vi "Variable Graphing.vi"(0 "Tree Refnum":refnum<vi>) -> ()   [LabVIEW 2017]
uses:
  <vilib>/Utility/miscctls.llb/LVRangeTypeDef.ctl
  <vilib>/Platform/TimedLoop/XDataNode/timing_clust.ctl
  <vilib>/Platform/TimedLoop/XDataNode/nitl_modes.ctl
  <vilib>/Platform/TimedLoop/XDataNode/wakeup.ctl
  <vilib>/Rock Robotics/Network Tables/NT Read Number.vi
  <vilib>/Rock Robotics/Network Tables/NT Write Number.vi
  <vilib>/Rock Robotics/Network Tables/NT Write Boolean.vi
  <vilib>/platform/TimedLoop/XDataNode/XDataNode.xnode
  <vilib>/Platform/TimedLoop/XDataNode/XDNodeRunTimeDep.lvlib
panel:
  in  "Camera Tab":enum32{"Graphs Setup", "PID Test", "Variables"}(tab)
  in  "Graph 2 Variable Selection":T1
  in  "Graph 1 Variable Selection":T2
  in  "Graph Include Filter":string[](array[string])
  in  "Graph Exclude Filter":string[](array[string])
  in  "Chart Update Rate Samples":i32=10
  in  "Waveform Depth Samples":i32=6000
  out "Chart":waveform(dbl)[](graph)
  out "Chart 2":waveform(dbl)[](graph)
  out "Samples":i32
  in  "Reset":bool
  in  "Pause":bool
  in  "Talon Performance Values":u16(ring) items=["/Talons/1/Bus Voltage", "/Talons/1/Closed Loop Error", "/Talons/1/Error Derivative", "/Talons/1/Integral Acummulator", "/Talons/1/Output Current", "/Talons/1/Output Voltage", "/Talons/1/Percent Output", "/Talons/1/Position", "/Talons/1/Velocity", "/Talons/1/pid:0/D", "/Talons/1/pid:0/FF", "/Talons/1/pid:0/I", "/Talons/1/pid:0/IZone", "/Talons/1/pid:0/P", "/Talons/1/pid:1/D", "/Talons/1/pid:1/FF", "/Talons/1/pid:1/I", "/Talons/1/pid:1/IZone", "/Talons/1/pid:1/P", "/Talons/2/Bus Voltage", "/Talons/2/Closed Loop Error", "/Talons/2/Error Derivative", "/Talons/2/Integral Acummulator", "/Talons/2/Output Current", "/Talons/2/Output Voltage", "/Talons/2/Percent Output", "/Talons/2/Position", "/Talons/2/Velocity", "/Talons/2/pid:0/D", "/Talons/2/pid:0/FF", "/Talons/2/pid:0/I", "/Talons/2/pid:0/IZone", "/Talons/2/pid:0/P", "/Talons/2/pid:1/D", "/Talons/2/pid:1/FF", "/Talons/2/pid:1/I", "/Talons/2/pid:1/IZone", "/Talons/2/pid:1/P", "/Talons/3/Bus Voltage", "/Talons/3/Closed Loop Error", "/Talons/3/Error Derivative", "/Talons/3/Integral Acummulator", "/Talons/3/Output Current", "/Talons/3/Output Voltage", "/Talons/3/Percent Output", "/Talons/3/Position", "/Talons/3/Velocity", "/Talons/3/pid:0/D", "/Talons/3/pid:0/FF", "/Talons/3/pid:0/I", "/Talons/3/pid:0/IZone", "/Talons/3/pid:0/P", "/Talons/3/pid:1/D", "/Talons/3/pid:1/FF", "/Talons/3/pid:1/I", "/Talons/3/pid:1/IZone", "/Talons/3/pid:1/P", "/Talons/4/Bus Voltage", "/Talons/4/Closed Loop Error", "/Talons/4/Error Derivative", "/Talons/4/Integral Acummulator", "/Talons/4/Output Current", "/Talons/4/Output Voltage", "/Talons/4/Percent Output", "/Talons/4/Position", "/Talons/4/Velocity", "/Talons/4/pid:0/D", "/Talons/4/pid:0/FF", "/Talons/4/pid:0/I", "/Talons/4/pid:0/IZone", "/Talons/4/pid:0/P", "/Talons/4/pid:1/D", "/Talons/4/pid:1/FF", "/Talons/4/pid:1/I", "/Talons/4/pid:1/IZone", "/Talons/4/pid:1/P"]
  in  "Talon Array":T3(array[cluster])
  in  "Run Selected":bool
  in  "Set Point":dbl
  in  "Read All":bool
  in  "Update\nSelected":bool
  in  "Talon ID Selector":u16(ring) items=["1", "2", "3", "4"]
  out "Chart 3":waveform(dbl)[](graph)
  in  "Pause PID":bool
  in  "Reset PID":bool
  out "Samples 2":i32
  in  "Waveform Depth Samples 2":i32=6000
  in  "Chart Update Rate Samples 2":i32=10
  out "Tree":string(tree)
  # "Graph 1"
  # "Graph 2"
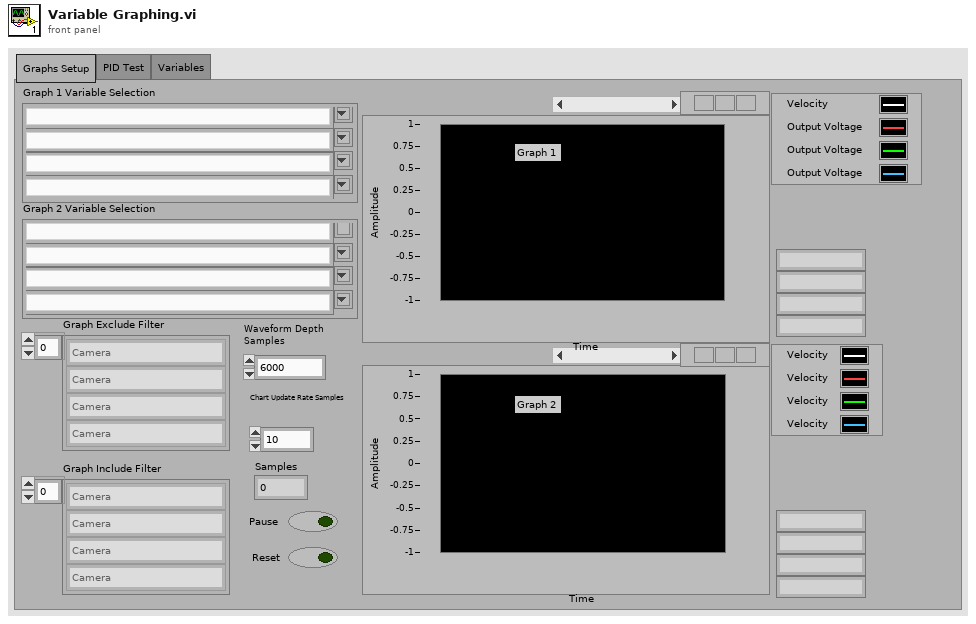
[diagram p1: front panel]
types:
  T1 = cluster{"Combo Box 5":string, "Combo Box 6":string, "Combo Box 7":string, "Combo Box 8":string}
  T2 = cluster{"Combo Box":string, "Combo Box 2":string, "Combo Box 3":string, "Combo Box 4":string}
  T3 = cluster{"P":dbl, "I":dbl, "D":dbl, "FF":dbl, "IZone":dbl, "RR":dbl, "Mode":dbl}[][]
  T4 = cluster{"P":dbl, "I":dbl, "D":dbl, "FF":dbl, "IZone":dbl, "RR":dbl, "Mode":dbl}
  T5 = typedef "LVRangeTypeDef.ctl" = cluster{"Minimum":dbl, "Maximum":dbl, "Increment":dbl, "Minor Increment":dbl, "Start":dbl}
  T6 = typedef "XDNodeRunTimeDep.lvlib/timing_clust.ctl" = cluster{"Expected End [f-1]":u64, "Actual End [f-1]":u64, "Finished Late? [f-1]":bool, "Expected End [i-1]":u64, "Actual End [i-1]":u64, "Finished Late? [i-1]":bool, "Expected Start [i]":u64, "Actual Start [i]":u64, "Expected Start [f]":u64, "Actual Start [f]":u64, "Source Name":string, "Structure Name":string, "Period":i64, "Deadline":i64, "Offset":i64, "Start":i64, "Priority":i32, "Timeout":i32, "Mode":T7, "Wakeup Reason":T8, "Error":errorcluster, "Source Type":string, "Secondary Source Type":string, "Global End Time":u64, "Global Start Time":u64, "Frame Duration":u64, "Iteration Duration":u64, "Assigned CPU":i32, "I/O Scan Engine Mode":u32}
  T7 = typedef "XDNodeRunTimeDep.lvlib/nitl_modes.ctl" = enum32{"No Change", "Process missed periods, maintain original phase", "Discard missed periods, maintain original phase", "Process missed periods, ignore original phase", "Discard missed periods, ignore original phase"}
  T8 = typedef "XDNodeRunTimeDep.lvlib/wakeup.ctl" = enum32{"Normal", "Aborted", "Asynchronous wakeup", "Timing source error", "Timed loop error", "Timeout"}
  T9 = cluster{"P":dbl, "I":dbl, "D":dbl, "FF":dbl, "IZone":dbl, "RR":dbl, "Mode":dbl}[]
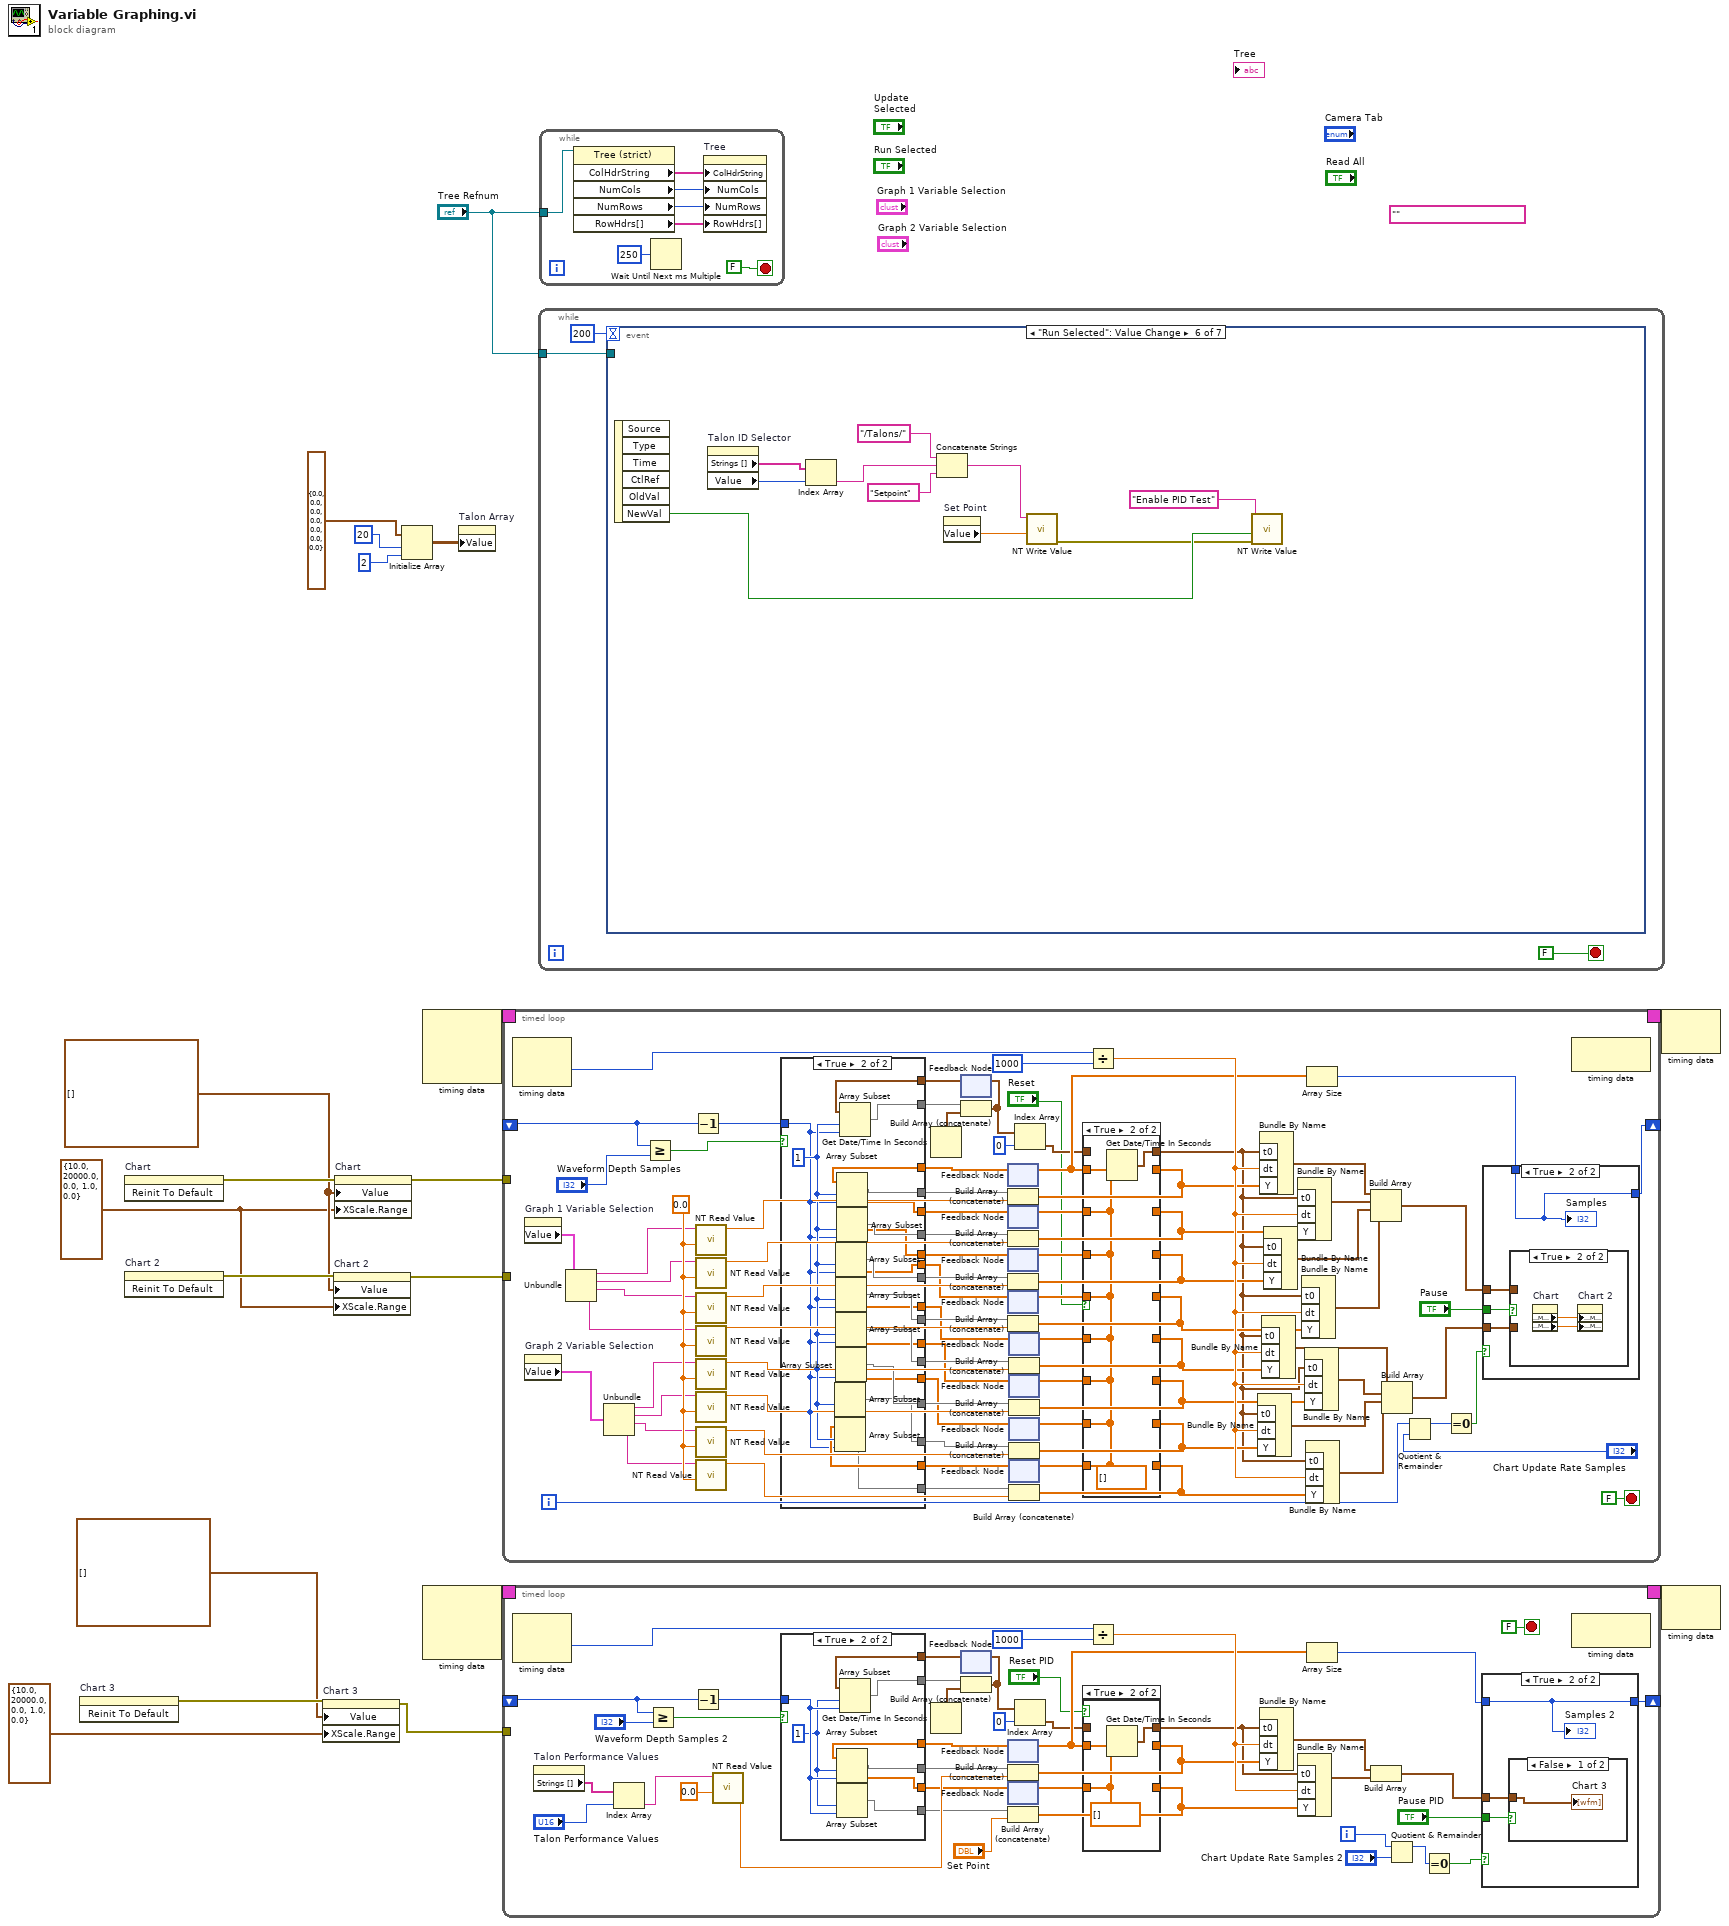
[diagram p0: block diagram]
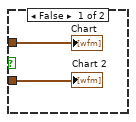
[diagram p8: hidden frame]
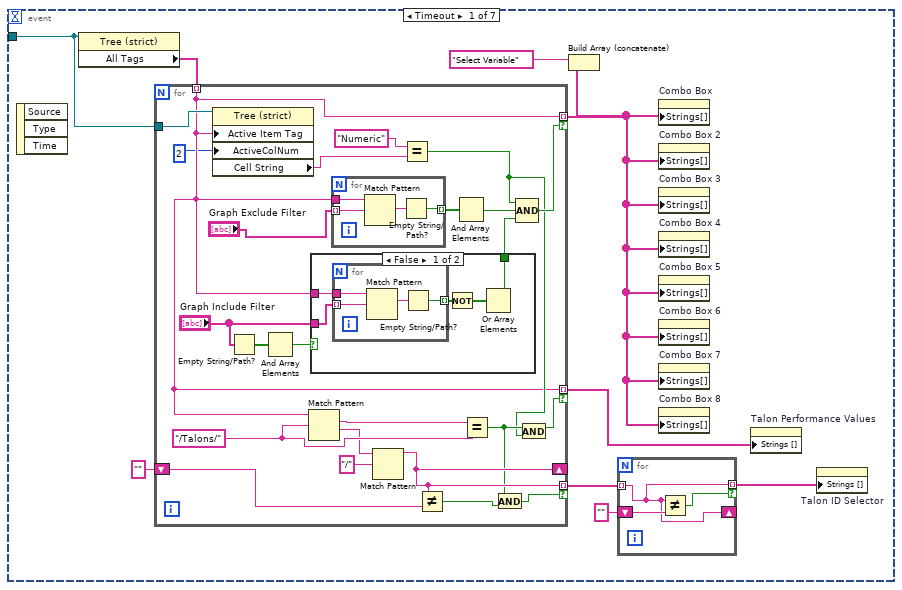
[diagram p10: hidden frame]
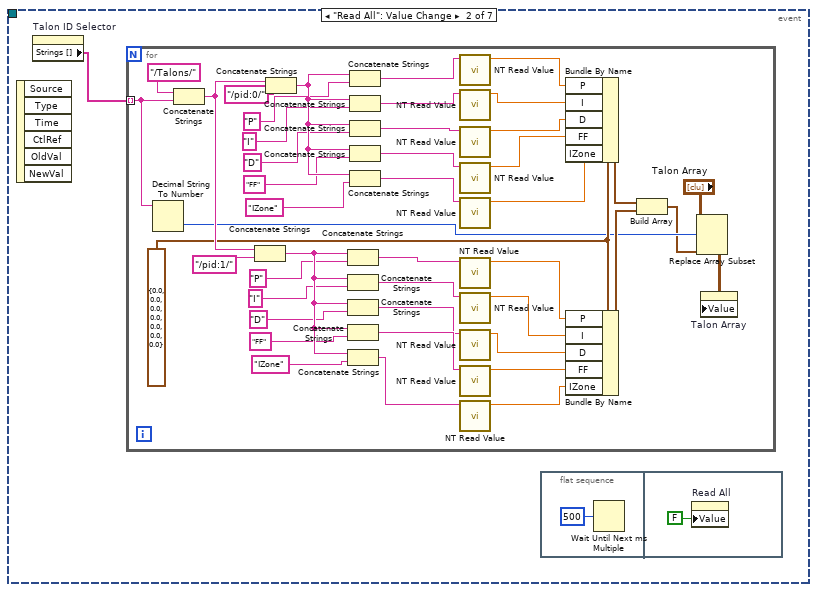
[diagram p12: hidden frame]
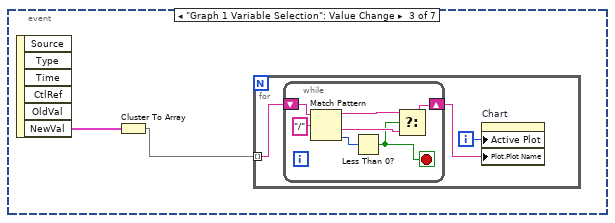
[diagram p13: hidden frame]
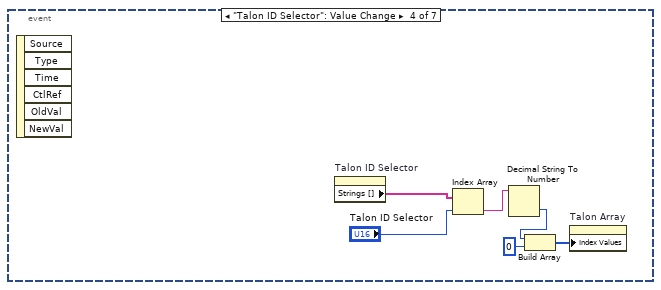
[diagram p14: hidden frame]
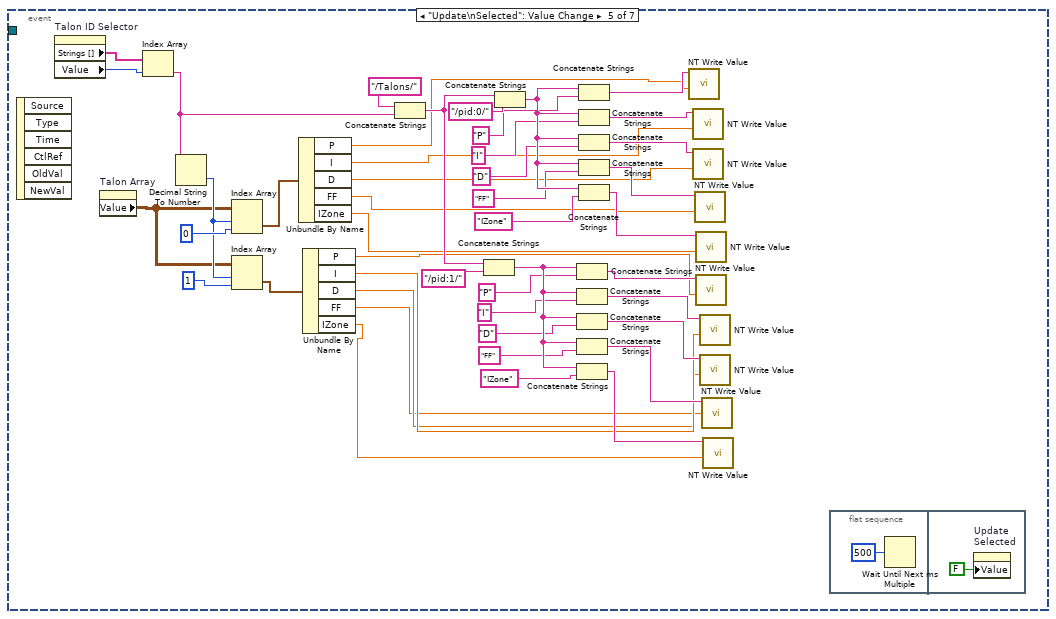
[diagram p15: hidden frame]
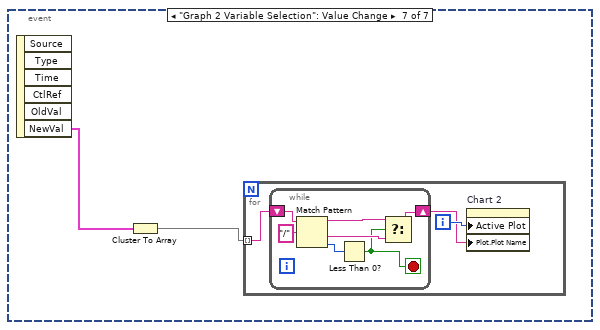
[diagram p16: hidden frame]
diagram:
  (unwired) "" ("Talon Performance Values")
  w14 = T5 {"Minimum"=10.0, "Maximum"=20000.0, "Increment"=0.0, "Minor Increment"=1.0, "Start"=0.0} ("X Scale.Range")
  w15 = waveform(dbl)[] []
  n1 = invoke on="Chart 3" class="WFChart (strict)" method="Reinit To Default"() -> (error out=w9:errorcluster)  [unwired: 3 in, 2 out]
  n2 = invoke on="Chart" class="WFChart (strict)" method="Reinit To Default"() -> (error out=w17:errorcluster)  [unwired: 3 in, 2 out]
  n3 = invoke on="Chart 2" class="WFChart (strict)" method="Reinit To Default"() -> (error out=w16:errorcluster)  [unwired: 3 in, 2 out]
  n4 = property on="Chart 3" class="WFChart (strict)"(error in=w9, "Value"=waveform(dbl)[] [], "XScale.Range"=T5 {"Minimum"=10.0, "Maximum"=20000.0, "Increment"=0.0, "Minor Increment"=1.0, "Start"=0.0} ("X Scale.Range")) -> (error out=w8:errorcluster)  [unwired: 1 in, 1 out]
  n5 = property on="Chart 2" class="WFChart (strict)"(error in=w16, "Value"=w15, "XScale.Range"=w14) -> (error out=w12:errorcluster)  [unwired: 1 in, 1 out]
  n6 = property on="Chart" class="WFChart (strict)"(error in=w17, "Value"=w15, "XScale.Range"=w14) -> (error out=w13:errorcluster)  [unwired: 1 in, 1 out]
  n7 = Initialize Array(T4 {"P"=0.0, "I"=0.0, "D"=0.0, "FF"=0.0, "IZone"=0.0, "RR"=0.0, "Mode"=0.0} ("PID Values"), 20 ("dimension size"), 2 ("dimension size")) -> (w1:T3)
  n8 = node-c288() -> (w19:T6)  [unwired: 3 in]
  n9 = node-c288() -> (w11:T6)  [unwired: 3 in]
  n10 = property on="Talon Array" class="Arr (strict)"("Value"=w1) -> ()  [unwired: 2 in, 2 out]
  n11 = timed-loop {
    timing: w19 -> [_]
    timing-out: [_] -> w18
    shift-right: [w21] -> _
    shift-left: _ -> [w20]
    tunnel: w13 -> [_]
    tunnel: w12 -> [_]
    i -> [w101]
    stop <- FALSE stop-if-true
    w98 = 0.0 ("Default Value")
    n12 = node-c288() -> (w97:i64)  [unwired: 1 in, 1 out]
    n13 = property on="Graph 1 Variable Selection" class="Clust (strict)"() -> ("Value"=w31:T2)  [unwired: 2 in, 2 out]
    n14 = property on="Graph 2 Variable Selection" class="Clust (strict)"() -> ("Value"=w29:T1)  [unwired: 2 in, 2 out]
    n15 = Unbundle(w31) -> ("Combo Box"=w35:string, "Combo Box 2"=w34:string, "Combo Box 3"=w33:string, "Combo Box 4"=w32:string)
    n16 = Unbundle(w29) -> ("Combo Box 5"=w30:string, "Combo Box 6"=w28:string, "Combo Box 7"=w27:string, "Combo Box 8"=w26:string)
    n17 = Greater Or Equal?(x=w20, y="Waveform Depth Samples") -> (x >= y?=w102:bool)
    n18 = Decrement(x=w20) -> (x-1=w95:i32)
    n19 = call-poly <vilib>:"NT Read Value.vi"("Default Value"=w98, "Name"=w35) -> ("Numeric"=w94:dbl)  [unwired: 8 in, 1 out]
    n20 = call-poly <vilib>:"NT Read Value.vi"("Default Value"=w98, "Name"=w34) -> ("Numeric"=w93:dbl)  [unwired: 8 in, 1 out]
    n21 = call-poly <vilib>:"NT Read Value.vi"("Default Value"=w98, "Name"=w33) -> ("Numeric"=w92:dbl)  [unwired: 8 in, 1 out]
    n22 = call-poly <vilib>:"NT Read Value.vi"("Default Value"=w98, "Name"=w32) -> ("Numeric"=w91:dbl)  [unwired: 8 in, 1 out]
    n23 = call-poly <vilib>:"NT Read Value.vi"("Default Value"=w98, "Name"=w30) -> ("Numeric"=w90:dbl)  [unwired: 8 in, 1 out]
    n24 = call-poly <vilib>:"NT Read Value.vi"("Default Value"=w98, "Name"=w28) -> ("Numeric"=w89:dbl)  [unwired: 8 in, 1 out]
    n25 = call-poly <vilib>:"NT Read Value.vi"("Default Value"=w98, "Name"=w27) -> ("Numeric"=w88:dbl)  [unwired: 8 in, 1 out]
    n26 = call-poly <vilib>:"NT Read Value.vi"("Default Value"=w98, "Name"=w26) -> ("Numeric"=w87:dbl)  [unwired: 8 in, 1 out]
    n27 = Get Date/Time In Seconds() -> (seconds since 1Jan1904=w42:timestamp)
    n28 = feedback #1() -> (w41:timestamp[])  [unwired: 1 in]
    n29 = feedback #2() -> (w75:dbl[])  [unwired: 1 in]
    n30 = feedback #3() -> (w73:dbl[])  [unwired: 1 in]
    n31 = feedback #4() -> (w71:dbl[])  [unwired: 1 in]
    n32 = feedback #5() -> (w69:dbl[])  [unwired: 1 in]
    n33 = feedback #6() -> (w67:dbl[])  [unwired: 1 in]
    n34 = feedback #7() -> (w65:dbl[])  [unwired: 1 in]
    n35 = feedback #8() -> (w63:dbl[])  [unwired: 1 in]
    n36 = feedback #9() -> (w61:dbl[])  [unwired: 1 in]
    n37 = case shown="True" w102 {
      tunnel: w95 -> [_ w135]
      tunnel: w75 -> [w132 w152]
      tunnel: [w132 w150] -> w74
      tunnel: w73 -> [w131 w149]
      tunnel: [w131 w148] -> w72
      tunnel: w71 -> [w130 w147]
      tunnel: [w130 w146] -> w70
      tunnel: w69 -> [w129 w145]
      tunnel: [w129 w144] -> w68
      tunnel: w67 -> [w128 w143]
      tunnel: [w128 w142] -> w66
      tunnel: w65 -> [w125 w141]
      tunnel: [w125 w140] -> w64
      tunnel: w63 -> [w126 w139]
      tunnel: [w126 w138] -> w62
      tunnel: w61 -> [w127 w137]
      tunnel: [w127 w136] -> w60
      tunnel: w41 -> [w124 w134]
      tunnel: [w124 w133] -> w40
      frame False {
      }
      frame True {
        w151 = 1 ("index")
        n38 = Array Subset(array=w139, index=w151, length=w135) -> (w138:dbl[])
        n39 = Array Subset(array=w137, index=w151, length=w135) -> (w136:dbl[])
        n40 = Array Subset(array=w147, index=w151, length=w135) -> (w146:dbl[])
        n41 = Array Subset(array=w145, index=w151, length=w135) -> (w144:dbl[])
        n42 = Array Subset(array=w143, index=w151, length=w135) -> (w142:dbl[])
        n43 = Array Subset(array=w141, index=w151, length=w135) -> (w140:dbl[])
        n44 = Array Subset(array=w152, index=w151, length=w135) -> (w150:dbl[])
        n45 = Array Subset(array=w149, index=w151, length=w135) -> (w148:dbl[])
        n46 = Array Subset(array=w134, index=w151, length=w135) -> (w133:timestamp[])
      }
    }
    n47 = Build Array (concatenate)(w40, w42) -> (w39:timestamp[])
    n48 = feedback-in #1(w39) -> ()
    n49 = Build Array (concatenate)(w74, w94) -> (w59:dbl[])
    n50 = Build Array (concatenate)(w72, w93) -> (w57:dbl[])
    n51 = Build Array (concatenate)(w70, w92) -> (w55:dbl[])
    n52 = Build Array (concatenate)(w68, w91) -> (w53:dbl[])
    n53 = Build Array (concatenate)(w66, w90) -> (w51:dbl[])
    n54 = Build Array (concatenate)(w64, w89) -> (w49:dbl[])
    n55 = Build Array (concatenate)(w62, w88) -> (w47:dbl[])
    n56 = Build Array (concatenate)(w60, w87) -> (w45:dbl[])
    n57 = Index Array(array=w39, index=0) -> (element=w37:timestamp)
    n58 = case shown="True" "Reset" {
      tunnel: [w112 w114] -> w44
      tunnel: w59 -> [w112 _]
      tunnel: [w111 w114] -> w58
      tunnel: w57 -> [w111 _]
      tunnel: w55 -> [w110 _]
      tunnel: [w110 w114] -> w56
      tunnel: [w109 w114] -> w54
      tunnel: w53 -> [w109 _]
      tunnel: [w108 w114] -> w52
      tunnel: w51 -> [w108 _]
      tunnel: [w107 w114] -> w50
      tunnel: w49 -> [w107 _]
      tunnel: [w106 w114] -> w48
      tunnel: w47 -> [w106 _]
      tunnel: [w105 w114] -> w46
      tunnel: w45 -> [w105 _]
      tunnel: w37 -> [w104 _]
      tunnel: [w104 w113] -> w43
      frame False {
      }
      frame True {
        w114 = dbl[] []
        n59 = Get Date/Time In Seconds() -> (seconds since 1Jan1904=w113:timestamp)
      }
    }
    n60 = feedback-in #2(w44) -> ()
    n61 = feedback-in #3(w58) -> ()
    n62 = feedback-in #4(w56) -> ()
    n63 = feedback-in #5(w54) -> ()
    n64 = feedback-in #6(w52) -> ()
    n65 = feedback-in #7(w50) -> ()
    n66 = feedback-in #8(w48) -> ()
    n67 = feedback-in #9(w46) -> ()
    n68 = Divide(x=w97, y=i64 1000) -> (x/y=w82:dbl)
    n69 = Bundle By Name("t0"=w43, "dt"=w82, "Y"=w47) -> (w77:waveform(dbl))  [unwired: 1 in]
    n70 = Bundle By Name("t0"=w43, "dt"=w82, "Y"=w59) -> (w86:waveform(dbl))  [unwired: 1 in]
    n71 = Bundle By Name("t0"=w43, "dt"=w82, "Y"=w51) -> (w80:waveform(dbl))  [unwired: 1 in]
    n72 = Bundle By Name("t0"=w43, "dt"=w82, "Y"=w55) -> (w83:waveform(dbl))  [unwired: 1 in]
    n73 = Bundle By Name("t0"=w43, "dt"=w82, "Y"=w57) -> (w85:waveform(dbl))  [unwired: 1 in]
    n74 = Bundle By Name("t0"=w43, "dt"=w82, "Y"=w53) -> (w84:waveform(dbl))  [unwired: 1 in]
    n75 = Bundle By Name("t0"=w43, "dt"=w82, "Y"=w49) -> (w78:waveform(dbl))  [unwired: 1 in]
    n76 = Bundle By Name("t0"=w43, "dt"=w82, "Y"=w45) -> (w79:waveform(dbl))  [unwired: 1 in]
    n77 = Array Size(array=w44) -> (size(s)=w36:i32)
    n78 = Build Array(w86, w85, w83, w84) -> (w81:waveform(dbl)[])
    n79 = Build Array(w80, w78, w77, w79) -> (w76:waveform(dbl)[])
    n80 = Quotient & Remainder(x=w101, y="Chart Update Rate Samples") -> (x-y*floor(x/y)=w100:i32)  [unwired: 1 out]
    n81 = Equal To 0?(x=w100) -> (x = 0?=w99:bool)
    n82 = case shown="True" w99 {
      tunnel: "Pause" -> [_ w119]
      tunnel: w81 -> [_ w118]
      tunnel: w76 -> [_ w117]
      tunnel: w36 -> [w115 w116]
      tunnel: [w115 w116] -> w21
      frame False {
      }
      frame True {
        n83 = case shown="True" w119 {
          tunnel: w118 -> [w121 _]
          tunnel: w117 -> [w120 _]
          frame False {
            "Chart" <- w121
            "Chart 2" <- w120
          }
          frame True {
            n84 = property on="Chart" class="WFChart (strict)"() -> ("XScale.Minimum"=w122:dbl, "XScale.Maximum"=w123:dbl)  [unwired: 2 in, 2 out]
            n85 = property on="Chart 2" class="WFChart (strict)"("XScale.Minimum"=w122, "XScale.Maximum"=w123) -> ()  [unwired: 2 in, 2 out]
          }
        }
        "Samples" <- w116
      }
    }
    n86 = node-c288() -> ()  [unwired: 1 in, 1 out]
  }
  n87 = timed-loop {
    timing: w11 -> [_]
    timing-out: [_] -> w10
    shift-right: [w166] -> _
    shift-left: _ -> [w165]
    tunnel: w8 -> [_]
    i -> [w193]
    stop <- FALSE stop-if-true
    n88 = node-c288() -> (w189:i64)  [unwired: 1 in, 1 out]
    n89 = property on="Talon Performance Values" class="Ring (strict)"() -> ("Strings []"=w162:string[])  [unwired: 2 in, 2 out]
    n90 = Index Array(array=w162, index="Talon Performance Values") -> (element=w160:string)
    n91 = Greater Or Equal?(x=w165, y="Waveform Depth Samples 2") -> (x >= y?=w194:bool)
    n92 = Decrement(x=w165) -> (x-1=w187:i32)
    n93 = call-poly <vilib>:"NT Read Value.vi"("Default Value"=0.0, "Name"=w160) -> ("Numeric"=w186:dbl)  [unwired: 8 in, 1 out]
    n94 = Get Date/Time In Seconds() -> (seconds since 1Jan1904=w173:timestamp)
    n95 = feedback #10() -> (w172:timestamp[])  [unwired: 1 in]
    n96 = feedback #11() -> (w181:dbl[])  [unwired: 1 in]
    n97 = feedback #12() -> (w179:dbl[])  [unwired: 1 in]
    n98 = case shown="True" w194 {
      tunnel: w187 -> [_ w212]
      tunnel: w181 -> [w208 w216]
      tunnel: [w208 w215] -> w180
      tunnel: w179 -> [w207 w214]
      tunnel: [w207 w213] -> w178
      tunnel: w172 -> [w206 w211]
      tunnel: [w206 w210] -> w171
      frame False {
      }
      frame True {
        w209 = 1 ("index")
        n99 = Array Subset(array=w216, index=w209, length=w212) -> (w215:dbl[])
        n100 = Array Subset(array=w214, index=w209, length=w212) -> (w213:dbl[])
        n101 = Array Subset(array=w211, index=w209, length=w212) -> (w210:timestamp[])
      }
    }
    n102 = Build Array (concatenate)(w171, w173) -> (w170:timestamp[])
    n103 = feedback-in #10(w170) -> ()
    n104 = Build Array (concatenate)(w180, w186) -> (w177:dbl[])
    n105 = Build Array (concatenate)(w178, "Set Point") -> (w175:dbl[])
    n106 = Index Array(array=w170, index=0) -> (element=w168:timestamp)
    n107 = case shown="True" "Reset PID" {
      tunnel: [w198 w199] -> w174
      tunnel: w177 -> [w198 _]
      tunnel: [w197 w199] -> w176
      tunnel: w175 -> [w197 _]
      tunnel: w168 -> [w196 _]
      tunnel: [w196 w200] -> w157
      frame False {
      }
      frame True {
        w199 = dbl[] []
        n108 = Get Date/Time In Seconds() -> (seconds since 1Jan1904=w200:timestamp)
      }
    }
    n109 = feedback-in #11(w174) -> ()
    n110 = feedback-in #12(w176) -> ()
    n111 = Divide(x=w189, y=i64 1000) -> (x/y=w183:dbl)
    n112 = Bundle By Name("t0"=w157, "dt"=w183, "Y"=w177) -> (w185:waveform(dbl))  [unwired: 1 in]
    n113 = Bundle By Name("t0"=w157, "dt"=w183, "Y"=w175) -> (w184:waveform(dbl))  [unwired: 1 in]
    n114 = Array Size(array=w174) -> (size(s)=w167:i32)
    n115 = Build Array(w185, w184) -> (w182:waveform(dbl)[])
    n116 = Quotient & Remainder(x=w193, y="Chart Update Rate Samples 2") -> (x-y*floor(x/y)=w192:i32)  [unwired: 1 out]
    n117 = Equal To 0?(x=w192) -> (x = 0?=w191:bool)
    n118 = case shown="True" w191 {
      tunnel: "Pause PID" -> [_ w204]
      tunnel: w182 -> [_ w203]
      tunnel: w167 -> [w201 w202]
      tunnel: [w201 w202] -> w166
      frame False {
      }
      frame True {
        n119 = case shown="False" w204 {
          tunnel: w203 -> [w205 _]
          frame False {
            "Chart 3" <- w205
          }
          frame True {
          }
        }
        "Samples 2" <- w202
      }
    }
    n120 = node-c288() -> ()  [unwired: 1 in, 1 out]
  }
  n121 = while {
    tunnel: "Tree Refnum" -> [w220]
    stop <- FALSE stop-if-true
    n122 = event shown="[5] \"Run Selected\": Value Change" {
      selector: _ -> [_ _ _ _ _ _ _]
      dyn-events: _ -> [_ _ _ _ _ _ _]
      timeout: 200 -> [_ _ _ _ _ _ _]
      tunnel: w220 -> [w227 _ _ _ _ _ _]
      event Timeout {
        n123 = event-data() -> ()  [unwired: 1 in, 3 out]
        n124 = property class="Tree (strict)"(reference=w227) -> ("All Tags"=w226:string[])  [unwired: 1 in, 2 out]
        n125 = for {
          tunnel: w226 -> [w237] mode=indexing
          tunnel: [w237] -> w231 mode=indexing if=w254
          tunnel: [w237] -> w229 mode=indexing if=w240
          tunnel: [w245] -> w225 mode=indexing if=w242
          shift-right: [w245] -> _
          shift-left: "" -> [w244]
          tunnel: w227 -> [w238]
          w249 = "/Talons/" ("Graph Include Filter 2")
          n126 = property class="Tree (strict)"(reference=w238, "Active Item Tag"=w237, "ActiveColNum"=2 ("Active Cell:Active Column Number")) -> ("Cell String"=w235:string)  [unwired: 1 in, 2 out]
          n127 = Empty String/Path?(string/path="Graph Include Filter") -> (empty?=w253:bool[])
          n128 = And Array Elements(Boolean array=w253) -> (logical AND=w252:bool)
          n129 = Match Pattern(string=w237, regular expression=w249) -> (match substring=w248:string, after substring=w246:string)  [unwired: 1 in, 2 out]
          n130 = case shown="False" w252 {
            selector: w252 -> [_ w268]
            tunnel: w237 -> [w261 _]
            tunnel: [w260 w268] -> w255
            tunnel: "Graph Include Filter" -> [w259 _]
            frame False {
              n131 = for {
                tunnel: [w267] -> w262 mode=indexing
                tunnel: w259 -> [w265] mode=indexing
                tunnel: w261 -> [w264]
                n132 = Match Pattern(string=w264, regular expression=w265) -> (match substring=w266:string)  [unwired: 1 in, 3 out]
                n133 = Empty String/Path?(string/path=w266) -> (empty?=w267:bool)
              }
              n134 = Not(x=w262) -> (.not. x?=w263:bool[])
              n135 = Or Array Elements(Boolean array=w263) -> (logical OR=w260:bool)
            }
            frame True {
            }
          }
          n136 = for {
            tunnel: "Graph Exclude Filter" -> [w272] mode=indexing
            tunnel: w237 -> [w270]
            tunnel: [w271] -> w257 mode=indexing
            n137 = Match Pattern(string=w270, regular expression=w272) -> (match substring=w269:string)  [unwired: 1 in, 3 out]
            n138 = Empty String/Path?(string/path=w269) -> (empty?=w271:bool)
          }
          n139 = Match Pattern(string=w246, regular expression="/") -> (before substring=w245:string)  [unwired: 1 in, 3 out]
          n140 = Equal?(x="Numeric" ("y"), y=w235) -> (x = y?=w239:bool)
          n141 = Not Equal?(x=w245, y=w244) -> (x != y?=w243:bool)
          n142 = And Array Elements(Boolean array=w257) -> (logical AND=w256:bool)
          n143 = Equal?(x=w248, y=w249) -> (x = y?=w241:bool)
          n144 = And(x=w241, y=w243) -> (x .and. y?=w242:bool)
          n145 = Compound Arithmetic op=AND(w239, w256, w255) -> (w254:bool)
          n146 = And(x=w241, y=w239) -> (x .and. y?=w240:bool)
        }
        n147 = Build Array (concatenate)("Select Variable", w231) -> ()  [unwired: 1 out]
        n148 = for {
          tunnel: w225 -> [w233] mode=indexing
          shift-right: [w233] -> _
          shift-left: "" -> [w234]
          tunnel: [w233] -> w223 mode=indexing if=w232
          n149 = Not Equal?(x=w233, y=w234) -> (x != y?=w232:bool)
        }
        n150 = property on="Combo Box" class="CmbBox"("Strings[]"=w231) -> ()  [unwired: 2 in, 2 out]
        n151 = property on="Combo Box 2" class="CmbBox"("Strings[]"=w231) -> ()  [unwired: 2 in, 2 out]
        n152 = property on="Combo Box 3" class="CmbBox"("Strings[]"=w231) -> ()  [unwired: 2 in, 2 out]
        n153 = property on="Combo Box 4" class="CmbBox"("Strings[]"=w231) -> ()  [unwired: 2 in, 2 out]
        n154 = property on="Combo Box 5" class="CmbBox"("Strings[]"=w231) -> ()  [unwired: 2 in, 2 out]
        n155 = property on="Combo Box 6" class="CmbBox"("Strings[]"=w231) -> ()  [unwired: 2 in, 2 out]
        n156 = property on="Combo Box 7" class="CmbBox"("Strings[]"=w231) -> ()  [unwired: 2 in, 2 out]
        n157 = property on="Combo Box 8" class="CmbBox"("Strings[]"=w231) -> ()  [unwired: 2 in, 2 out]
        n158 = property on="Talon Performance Values" class="Ring (strict)"("Strings []"=w229) -> ()  [unwired: 2 in, 2 out]
        n159 = property on="Talon ID Selector" class="Ring (strict)"("Strings []"=w223) -> ()  [unwired: 2 in, 2 out]
      }
      event "Read All": Value Change {
        n160 = event-data() -> ()  [unwired: 1 in, 6 out]
        n161 = property on="Talon ID Selector" class="Ring (strict)"() -> ("Strings []"=w273:string[])  [unwired: 2 in, 2 out]
        n162 = for {
          tunnel: w273 -> [w318] mode=indexing
          w294 = T4 {"P"=0.0, "I"=0.0, "D"=0.0, "FF"=0.0, "IZone"=0.0, "RR"=0.0, "Mode"=0.0} ("PID Values")
          n163 = Decimal String To Number(string=w318) -> (number=w292:i32)  [unwired: 2 in, 1 out]
          n164 = Concatenate Strings("/Talons/" ("string"), w318) -> (w317:string)
          n165 = Concatenate Strings(w317, "/pid:1/") -> (w313:string)
          n166 = Concatenate Strings(w317, "/pid:0/") -> (w314:string)
          n167 = Concatenate Strings(w313, "P") -> (w298:string)
          n168 = Concatenate Strings(w313, "I") -> (w299:string)
          n169 = Concatenate Strings(w313, "D") -> (w300:string)
          n170 = Concatenate Strings(w313, "FF") -> (w301:string)
          n171 = Concatenate Strings(w313, "IZone") -> (w302:string)
          n172 = Concatenate Strings(w314, "P") -> (w280:string)
          n173 = Concatenate Strings(w314, "I") -> (w279:string)
          n174 = Concatenate Strings(w314, "D") -> (w278:string)
          n175 = Concatenate Strings(w314, "FF") -> (w277:string)
          n176 = Concatenate Strings(w314, "IZone") -> (w276:string)
          n177 = call-poly <vilib>:"NT Read Value.vi"("Name"=w280) -> ("Numeric"=w290:dbl)  [unwired: 9 in, 1 out]
          n178 = call-poly <vilib>:"NT Read Value.vi"("Name"=w279) -> ("Numeric"=w289:dbl)  [unwired: 9 in, 1 out]
          n179 = call-poly <vilib>:"NT Read Value.vi"("Name"=w278) -> ("Numeric"=w288:dbl)  [unwired: 9 in, 1 out]
          n180 = call-poly <vilib>:"NT Read Value.vi"("Name"=w277) -> ("Numeric"=w287:dbl)  [unwired: 9 in, 1 out]
          n181 = call-poly <vilib>:"NT Read Value.vi"("Name"=w276) -> ("Numeric"=w286:dbl)  [unwired: 9 in, 1 out]
          n182 = call-poly <vilib>:"NT Read Value.vi"("Name"=w298) -> ("Numeric"=w285:dbl)  [unwired: 9 in, 1 out]
          n183 = call-poly <vilib>:"NT Read Value.vi"("Name"=w299) -> ("Numeric"=w284:dbl)  [unwired: 9 in, 1 out]
          n184 = call-poly <vilib>:"NT Read Value.vi"("Name"=w300) -> ("Numeric"=w283:dbl)  [unwired: 9 in, 1 out]
          n185 = call-poly <vilib>:"NT Read Value.vi"("Name"=w301) -> ("Numeric"=w282:dbl)  [unwired: 9 in, 1 out]
          n186 = call-poly <vilib>:"NT Read Value.vi"("Name"=w302) -> ("Numeric"=w281:dbl)  [unwired: 9 in, 1 out]
          n187 = Bundle By Name(cluster=w294, "P"=w290, "I"=w289, "D"=w288, "FF"=w287, "IZone"=w286) -> (w297:T4)
          n188 = Bundle By Name(cluster=w294, "P"=w285, "I"=w284, "D"=w283, "FF"=w282, "IZone"=w281) -> (w296:T4)
          n189 = Build Array(w297, w296) -> (w291:T9)
          n190 = Replace Array Subset(array="Talon Array", new element=w291, index (row)=w292) -> (w293:T3)  [unwired: 1 in]
          n191 = property on="Talon Array" class="Arr (strict)"("Value"=w293) -> ()  [unwired: 2 in, 2 out]
        }
        n192 = flat-sequence {
          frame #0 {
            n193 = Wait Until Next ms Multiple(millisecond multiple=u32 500) -> ()  [unwired: 1 out]
          }
          frame #1 {
            n194 = property on="Read All" class="Bool (strict)"("Value"=FALSE ("Read All")) -> ()  [unwired: 2 in, 2 out]
          }
        }
      }
      event "Graph 1 Variable Selection": Value Change {
        n195 = event-data() -> ("NewVal"=w320:T2)  [unwired: 1 in, 5 out]
        n196 = Cluster To Array(cluster=w320) -> (array=w321:string[])
        n197 = for {
          tunnel: w321 -> [w323] mode=indexing
          i -> [w324]
          n198 = while {
            shift-right: [w328] -> w322
            shift-left: w323 -> [w331]
            stop <- w325 stop-if-true
            n199 = Match Pattern(string=w331, regular expression="/" ("search string/char (-)")) -> (before substring=w327:string, after substring=w326:string, offset past match=w329:i32)  [unwired: 1 in, 1 out]
            n200 = Less Than 0?(x=w329) -> (x < 0?=w325:bool)
            n201 = Select(t=w327, s=w325, f=w326) -> (s? t:f=w328:string)
          }
          n202 = property on="Chart" class="WFChart (strict)"("Active Plot"=w324, "Plot.Plot Name"=w322) -> ()  [unwired: 2 in, 2 out]
        }
      }
      event "Talon ID Selector": Value Change {
        n203 = event-data() -> ()  [unwired: 1 in, 6 out]
        n204 = property on="Talon ID Selector" class="Ring (strict)"() -> ("Strings []"=w335:string[])  [unwired: 2 in, 2 out]
        n205 = Index Array(array=w335, index="Talon ID Selector") -> (element=w332:string)
        n206 = Decimal String To Number(string=w332) -> (number=w333:i32)  [unwired: 2 in, 1 out]
        n207 = Build Array(w333, u16 0 ("element")) -> (w336:i32[])
        n208 = property on="Talon Array" class="Arr (strict)"("Index Values"=w336) -> ()  [unwired: 2 in, 2 out]
      }
      event "Update\nSelected": Value Change {
        n209 = event-data() -> ()  [unwired: 1 in, 6 out]
        n210 = property on="Talon ID Selector" class="Ring (strict)"() -> ("Strings []"=w382:string[], "Value"=w381:u16)  [unwired: 2 in, 2 out]
        n211 = property on="Talon Array" class="Arr (strict)"() -> ("Value"=w357:T3)  [unwired: 2 in, 2 out]
        n212 = Index Array(array=w382, index=w381) -> (element=w363:string)
        n213 = Decimal String To Number(string=w363) -> (number=w361:i32)  [unwired: 2 in, 1 out]
        n214 = Index Array(array=w357, index (row)=w361, index (col)=0 ("element")) -> (element=w359:T4)
        n215 = Index Array(array=w357, index (row)=w361, index (col)=1 ("element")) -> (element=w358:T4)
        n216 = Unbundle By Name(w359) -> ("P"=w347:dbl, "I"=w346:dbl, "D"=w345:dbl, "FF"=w344:dbl, "IZone"=w343:dbl)
        n217 = Unbundle By Name(w358) -> ("P"=w342:dbl, "I"=w341:dbl, "D"=w340:dbl, "FF"=w339:dbl, "IZone"=w338:dbl)
        n218 = Concatenate Strings("/Talons/" ("string"), w363) -> (w379:string)
        n219 = Concatenate Strings(w379, "/pid:1/") -> (w375:string)
        n220 = Concatenate Strings(w379, "/pid:0/") -> (w376:string)
        n221 = Concatenate Strings(w375, "P") -> (w356:string)
        n222 = Concatenate Strings(w375, "I") -> (w355:string)
        n223 = Concatenate Strings(w375, "D") -> (w354:string)
        n224 = Concatenate Strings(w375, "FF") -> (w353:string)
        n225 = Concatenate Strings(w375, "IZone") -> (w352:string)
        n226 = Concatenate Strings(w376, "P") -> (w364:string)
        n227 = Concatenate Strings(w376, "I") -> (w348:string)
        n228 = Concatenate Strings(w376, "D") -> (w349:string)
        n229 = Concatenate Strings(w376, "FF") -> (w350:string)
        n230 = Concatenate Strings(w376, "IZone") -> (w351:string)
        n231 = call-poly <vilib>:"NT Write Value.vi"("Numeric"=w347, "Name"=w364) -> ()  [unwired: 9 in, 1 out]
        n232 = call-poly <vilib>:"NT Write Value.vi"("Numeric"=w346, "Name"=w348) -> ()  [unwired: 9 in, 1 out]
        n233 = call-poly <vilib>:"NT Write Value.vi"("Numeric"=w345, "Name"=w349) -> ()  [unwired: 9 in, 1 out]
        n234 = call-poly <vilib>:"NT Write Value.vi"("Numeric"=w344, "Name"=w350) -> ()  [unwired: 9 in, 1 out]
        n235 = call-poly <vilib>:"NT Write Value.vi"("Numeric"=w343, "Name"=w351) -> ()  [unwired: 9 in, 1 out]
        n236 = call-poly <vilib>:"NT Write Value.vi"("Numeric"=w342, "Name"=w356) -> ()  [unwired: 9 in, 1 out]
        n237 = call-poly <vilib>:"NT Write Value.vi"("Numeric"=w341, "Name"=w355) -> ()  [unwired: 9 in, 1 out]
        n238 = call-poly <vilib>:"NT Write Value.vi"("Numeric"=w340, "Name"=w354) -> ()  [unwired: 9 in, 1 out]
        n239 = call-poly <vilib>:"NT Write Value.vi"("Numeric"=w339, "Name"=w353) -> ()  [unwired: 9 in, 1 out]
        n240 = call-poly <vilib>:"NT Write Value.vi"("Numeric"=w338, "Name"=w352) -> ()  [unwired: 9 in, 1 out]
        n241 = flat-sequence {
          frame #0 {
            n242 = Wait Until Next ms Multiple(millisecond multiple=u32 500) -> ()  [unwired: 1 out]
          }
          frame #1 {
            n243 = property on="Update\nSelected" class="Bool (strict)"("Value"=FALSE ("Update\nSelected")) -> ()  [unwired: 2 in, 2 out]
          }
        }
      }
      event "Run Selected": Value Change {
        n244 = event-data() -> ("NewVal"=w387:bool)  [unwired: 1 in, 5 out]
        n245 = property on="Talon ID Selector" class="Ring (strict)"() -> ("Strings []"=w393:string[], "Value"=w392:u16)  [unwired: 2 in, 2 out]
        n246 = Index Array(array=w393, index=w392) -> (element=w390:string)
        n247 = Concatenate Strings("/Talons/", w390, "Setpoint") -> (w388:string)
        n248 = property on="Set Point" class="DigNum (strict)"() -> ("Value"=w394:dbl)  [unwired: 2 in, 2 out]
        n249 = call-poly <vilib>:"NT Write Value.vi"("Numeric"=w394, "Name"=w388) -> ("error out"=w385:errorcluster)  [unwired: 9 in]
        n250 = call-poly <vilib>:"NT Write Value.vi"("error in"=w385, "Boolean"=w387, "Name"="Enable PID Test") -> ()  [unwired: 8 in, 1 out]
      }
      event "Graph 2 Variable Selection": Value Change {
        n251 = event-data() -> ("NewVal"=w395:T1)  [unwired: 1 in, 5 out]
        n252 = Cluster To Array(cluster=w395) -> (array=w396:string[])
        n253 = for {
          tunnel: w396 -> [w398] mode=indexing
          i -> [w399]
          n254 = while {
            shift-right: [w403] -> w397
            shift-left: w398 -> [w406]
            stop <- w400 stop-if-true
            n255 = Match Pattern(string=w406, regular expression="/" ("search string/char (-)")) -> (before substring=w402:string, after substring=w401:string, offset past match=w404:i32)  [unwired: 1 in, 1 out]
            n256 = Less Than 0?(x=w404) -> (x < 0?=w400:bool)
            n257 = Select(t=w402, s=w400, f=w401) -> (s? t:f=w403:string)
          }
          n258 = property on="Chart 2" class="WFChart (strict)"("Active Plot"=w399, "Plot.Plot Name"=w397) -> ()  [unwired: 2 in, 2 out]
        }
      }
    }
  }
  n259 = while {
    tunnel: "Tree Refnum" -> [w409]
    stop <- FALSE stop-if-true
    n260 = property class="Tree (strict)"(reference=w409) -> ("ColHdrString"=w410:string[], "NumCols"=w411:u32, "NumRows"=w412:u32, "RowHdrs[]"=w413:string[])  [unwired: 1 in, 2 out]
    n261 = Wait Until Next ms Multiple(millisecond multiple=u32 250) -> ()  [unwired: 1 out]
    n262 = property on="Tree" class="Tree (strict)"("ColHdrString"=w410, "NumCols"=w411, "NumRows"=w412, "RowHdrs[]"=w413) -> ()  [unwired: 2 in, 2 out]
  }
  n263 = node-c288(w18) -> ()  [unwired: 1 out]
  n264 = node-c288(w10) -> ()  [unwired: 1 out]
